vi "Graph_transform_rect.vi"(2 "rect in":T1, 3 "ref in":refnum<vi>) -> (0 "rect out":T1, 1 "ref out":refnum<vi>)   [LabVIEW 2010]
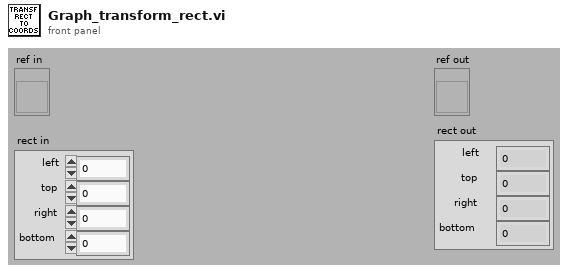
[diagram p1: front panel]
types:
  T1 = cluster{"left":i16, "top":i16, "right":i16, "bottom":i16}
  T2 = typedef "LVRectTypeDef.ctl" = cluster{"left":i16, "top":i16, "right":i16, "bottom":i16}
  T3 = typedef "LVPoint32TypeDef.ctl" = cluster{"Horizontal":i32, "Vertical":i32}
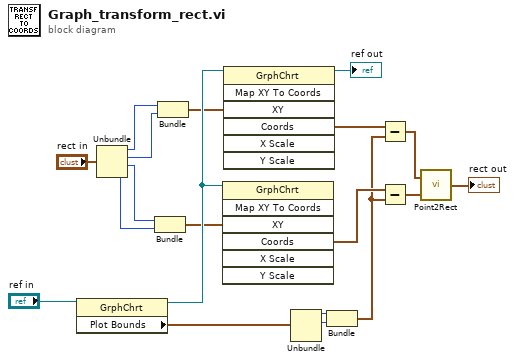
[diagram p0: block diagram]
diagram:
  n1 = property on="Property Node" class="GrphChrt"(reference="ref in") -> (reference out=w15:refnum<vi>, "Plot Bounds"=w10:T2)  [unwired: 1 in, 1 out]
  n2 = Unbundle("rect in") -> ("left"=w7:i16, "top"=w6:i16, "right"=w5:i16, "bottom"=w4:i16)
  n3 = Bundle("right"=w5, "bottom"=w4) -> (w2:cluster{"right":i16, "bottom":i16})  [unwired: 1 in]
  n4 = Bundle("left"=w7, "top"=w6) -> (w3:cluster{"left":i16, "top":i16})  [unwired: 1 in]
  n5 = invoke on="Invoke Node" class="GrphChrt" method="Map XY To Coords"(reference=w15, "XY"=w2) -> ("Coords"=w16:T3)  [unwired: 5 in, 6 out]
  n6 = invoke on="Invoke Node" class="GrphChrt" method="Map XY To Coords"(reference=w15, "XY"=w3) -> (reference out=→"ref out":refnum<vi>, "Coords"=w19:T3)  [unwired: 5 in, 5 out]
  n7 = Unbundle(w10) -> ("left"=w13:i16, "top"=w12:i16)  [unwired: 2 out]
  n8 = Bundle("left"=w13, "top"=w12) -> (w14:cluster{"left":i16, "top":i16})  [unwired: 1 in]
  n9 = Subtract(x=w19, y=w14) -> (x-y=w18:T3)
  n10 = Subtract(x=w16, y=w14) -> (x-y=w17:T3)
  n11 = call <vilib>:"Point2Rect.vi"("point b"=w17, "point a"=w18) -> ("rect"=→"rect out":T1)
